vi "Engine Out - Spark.vi"(0 "Spark Timings (DBTDC)":sgl[](array[numeric]), 1 "Spark Dwells (ms)":sgl[](array[numeric])) -> (11 "Spark 8":T1, 13 "Spark 7":T1, 14 "Spark 1":T1, 15 "Spark 2":T1, 16 "Spark 3":T1, 17 "Spark 4":T1, 18 "Spark 5":T1, 19 "Spark 6":T1)   [LabVIEW 2015, in "ECS-RT.lvlib"]
uses:
  ECS-RT.lvlib
  Typedefs/Raw Outputs/ESTTL.ctl
  ECS-Shared.lvlib
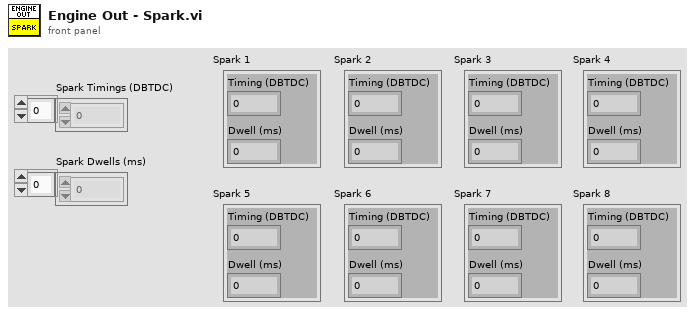
[diagram p1: front panel]
types:
  T1 = typedef "ECS-Shared.lvlib/ESTTL.ctl" = cluster{"Timing (DBTDC)":sgl, "Dwell (ms)":sgl}
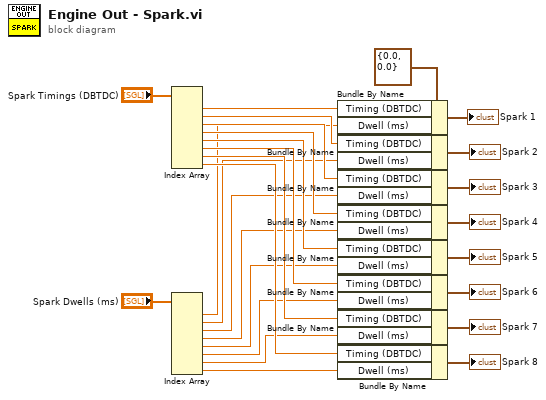
[diagram p0: block diagram]
diagram:
  w27 = T1 {"Timing (DBTDC)"=0.0, "Dwell (ms)"=0.0} ("Spark")
  n1 = Index Array(array="Spark Timings (DBTDC)") -> (element #1=w16:sgl, element #2=w15:sgl, element #3=w14:sgl, element #4=w13:sgl, element #5=w12:sgl, element #6=w11:sgl, element #7=w10:sgl, element #8=w9:sgl)  [unwired: 8 in]
  n2 = Index Array(array="Spark Dwells (ms)") -> (element #1=w1:sgl, element #2=w2:sgl, element #3=w3:sgl, element #4=w4:sgl, element #5=w5:sgl, element #6=w6:sgl, element #7=w7:sgl, element #8=w8:sgl)  [unwired: 8 in]
  n3 = Bundle By Name(cluster=w27, "Timing (DBTDC)"=w16, "Dwell (ms)"=w1) -> (→"Spark 1":T1)
  n4 = Bundle By Name(cluster=w27, "Timing (DBTDC)"=w15, "Dwell (ms)"=w2) -> (→"Spark 2":T1)
  n5 = Bundle By Name(cluster=w27, "Timing (DBTDC)"=w14, "Dwell (ms)"=w3) -> (→"Spark 3":T1)
  n6 = Bundle By Name(cluster=w27, "Timing (DBTDC)"=w13, "Dwell (ms)"=w4) -> (→"Spark 4":T1)
  n7 = Bundle By Name(cluster=w27, "Timing (DBTDC)"=w12, "Dwell (ms)"=w5) -> (→"Spark 5":T1)
  n8 = Bundle By Name(cluster=w27, "Timing (DBTDC)"=w11, "Dwell (ms)"=w6) -> (→"Spark 6":T1)
  n9 = Bundle By Name(cluster=w27, "Timing (DBTDC)"=w10, "Dwell (ms)"=w7) -> (→"Spark 7":T1)
  n10 = Bundle By Name(cluster=w27, "Timing (DBTDC)"=w9, "Dwell (ms)"=w8) -> (→"Spark 8":T1)
